vi "Find Average Center.vi"(5 "Position":i32, 7 "Tray Number":i32, 9 "XYZTheta":dbl[](array[numeric]), 11 "Gantry In":refnum<k24>) -> (1 "XYZTheta":dbl[](array[numeric]) format="%.6g", 3 "Gantry Out":refnum<k24>)   [LabVIEW 2021, in "Component Tray.lvclass"]
uses:
  Component Tray.lvclass
  Find Component.ctl
  Controller/Camera/Machine Vision.ctl
  C:/Program Files (x86)/Aerotech/A3200/LabVIEW/2010/Bin/Aerotech.A3200.dll
  Program Files (x86)/Aerotech/A3200/LabVIEW/2010/Bin/Aerotech.A3200.dll
  Controller/Camera/Image processing.ctl
  Controller/Camera/Camera settings.ctl
  Controller/Camera/Material.ctl
  Controller/Camera/Edmund Optics/Edmund Optics.lvclass
  C:/Users/HEP/Documents/GitHub/UCSB-Gantry-HEP/Classes/Controller/Camera/Camera.lvclass
  Program Files (x86)/National Instruments/LabVIEW 2021/examples/Connectivity/Python/support/PythonVersionsEnum.ctl
  Controller/Camera/Camera.lvclass
  Controller/Motion/A3200/A3200.lvclass
  Controller/Motion/Motion.lvclass
panel:
  out "Program Stopped":bool
  out "XY Graph":cluster{"X":dbl, "Y":dbl}[](graph)
  out "Sensor ID Location":dbl[](array[numeric])
  in  "Go to Sensor ID":bool
  out "CH1 Location":dbl[](array[numeric])
  in  "Verify CH1":bool
  out "CH1 correct?":bool
  in  "Go to CH1":bool
  in  "Focus step size":dbl format="%#_13g"
  in  "number of focus steps":i32
  out "Average Strength":dbl
  in  "Focus":bool
  in  "Material":T1
  out "All fiducials recorded":bool
  in  "Override presets":bool
  in  "Camera settings":T2={"Gamma"=1.6, "Gain"=0, "Sharpness"=0, "Contrast"=0.0, "Exposure"=0.0078125} {"Exposure" min=0.000244140625 max=0.5 scale=0.0002..0.5; "Contrast" min=0.0 max=1.0 scale=0.001..1.0; "Sharpness" min=0 max=2 step=1 scale=0.0..2.0; "Gain" min=0 max=100 step=1 scale=0.1..100.0; "Gamma" min=0.01 max=10.0 scale=0.01..10.0}
  in  "Image processing":T3={"Brightness"=128.0, "Contrast"=45.0, "Gamma"=1.0471123} {"Brightness" scale=0.0..400.0; "Contrast" scale=0.0..90.0; "Gamma" scale=0.005..5.0}
  in  "Machine Vision":T4
  out "Gantry":dbl[](array[numeric]) format="%.6g"
  out "Sum":dbl[](array[numeric]) format="%.6g"
  out "CH111/FD3 XY":dbl[](array[numeric]) format="%.6g"
  out "CH95/FD3 XY":dbl[](array[numeric]) format="%.6g"
  out "CH96/FD6 XY":dbl[](array[numeric]) format="%.6g"
  out "CH81/FD6 XY":dbl[](array[numeric]) format="%.6g"
  in  "Record CH95/FD3":bool
  in  "Record CH111/FD3":bool
  in  "Record CH96/FD6":bool
  in  "Record CH81/FD6":bool
  in  "Go to CH111/FD3":bool
  in  "Go to CH95/FD3":bool
  in  "Go to CH96/FD6":bool
  in  "Go to CH81/FD6":bool
  in  "Joystick":bool
  out "Camera":dbl[](array[numeric]) format="%.6g"
  in  "Go to Center":bool
  in  "Component":T5
  in  "Stop Program":bool
  out "Image":T6(plugin-control)
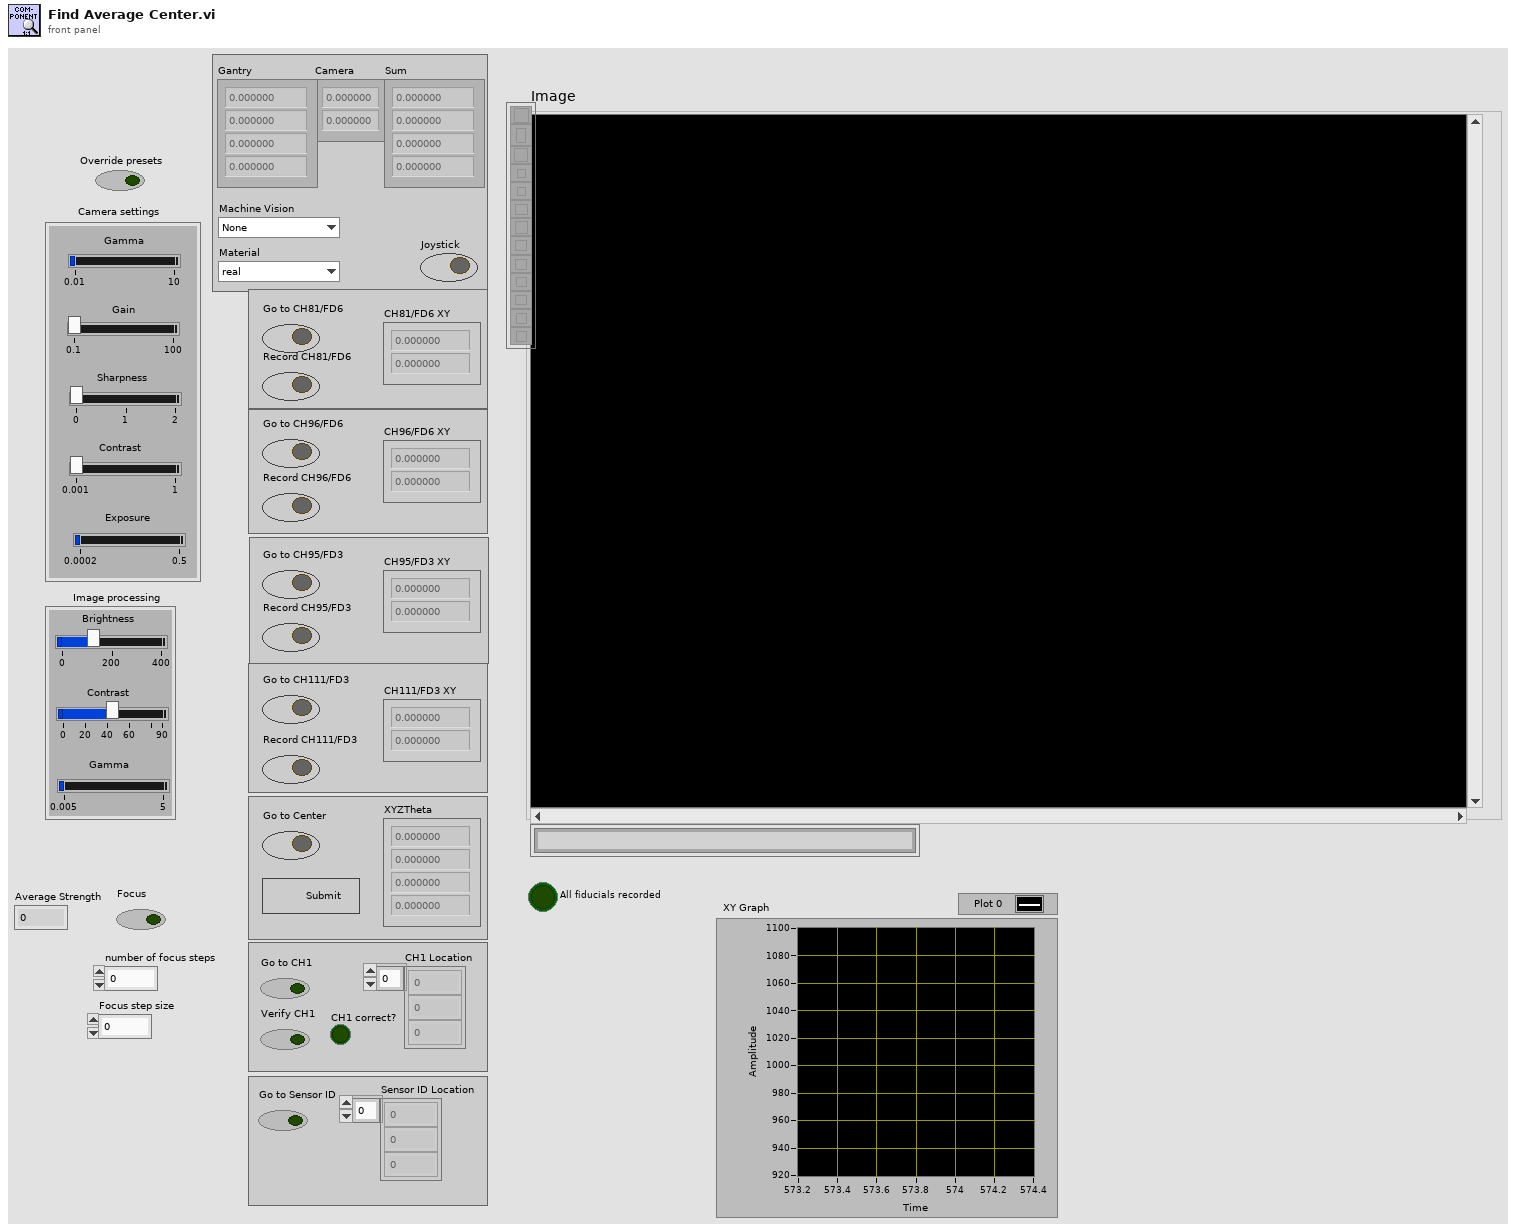
[diagram p1: front panel]
types:
  T1 = typedef "Camera.lvclass/Material.ctl" = enum16{"real", "dummy", "PETG"}
  T2 = typedef "Camera.lvclass/Camera settings.ctl" = cluster{"Gamma":dbl, "Gain":i64, "Sharpness":i64, "Contrast":dbl, "Exposure":dbl}
  T3 = typedef "Camera.lvclass/Image processing.ctl" = cluster{"Brightness":sgl, "Contrast":sgl, "Gamma":sgl}
  T4 = typedef "Camera.lvclass/Machine Vision.ctl" = enum16{"None", "Tray Fiducials", "HPK Silicon", "100um dot", "Hexaboard", "Corner (TL, BR)", "Corner (BL, TR)", "BP gold pad 1", "BP gold pad 2", "BP gold pad 3", "dummy sensor CH2", "dummy sensor CH7", "dummy sensor CH191", "dummy sensor CH197", "sensor box", "sensor circle", "PCB PETG CH2", "PCB PETG CH7", "PCB PETG CH191", "PCB PETG CH197"}
  T5 = typedef "Component Tray.lvclass/Find Component.ctl" = cluster{"New Fiducials":dbl[], "Past Fiducials":dbl[], "XYZTheta":dbl[], "Fiducials Path":path, "Position":i32, "CH1 Location":dbl[], "Sensor ID Location":dbl[]}
  T6 = typedef "IMAQ Image.ctl" = refnum<image>
  T7 = typedef "File Paths.ctl" = cluster{"Glue Pattern Folder":path, "Carrier Tray Folder":path, "Pick Up Tool Fixture Folder":path, "Components Folder":path, "Bellows Tool Offset.txt":path, "Pick Up Tool Offset.txt":path, "Dispense Tip Offset.txt":path, "Log Files":path, "Gantry Assembly Map.txt":path, "Syringe and offset map.txt":path, "Python DB Conn":path}
  T8 = typedef "PythonVersionsEnum.ctl" = enum16{"3.6", "3.7", "3.8", "3.9"}
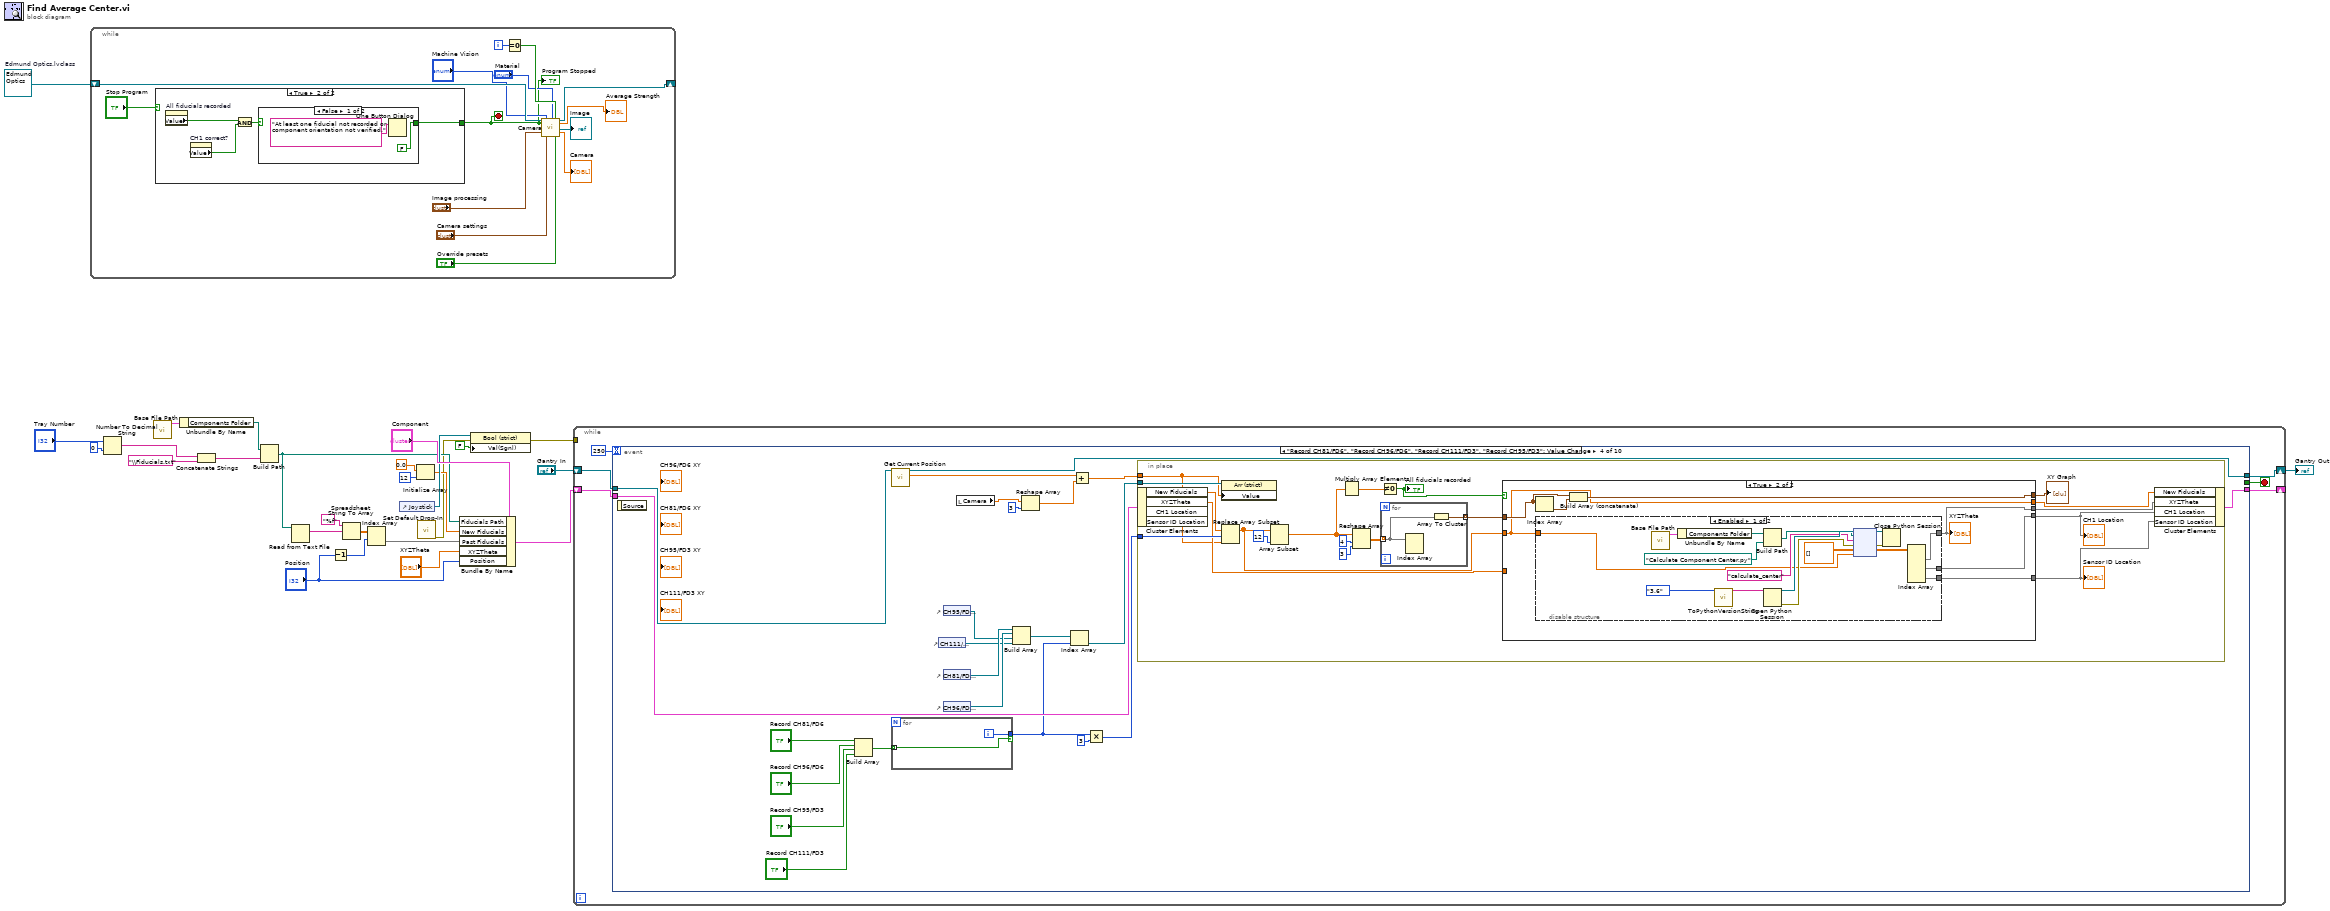
[diagram p0: block diagram]
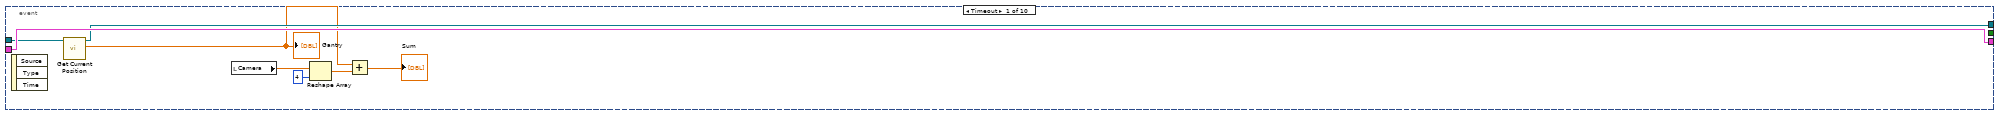
[diagram p2: hidden frame]
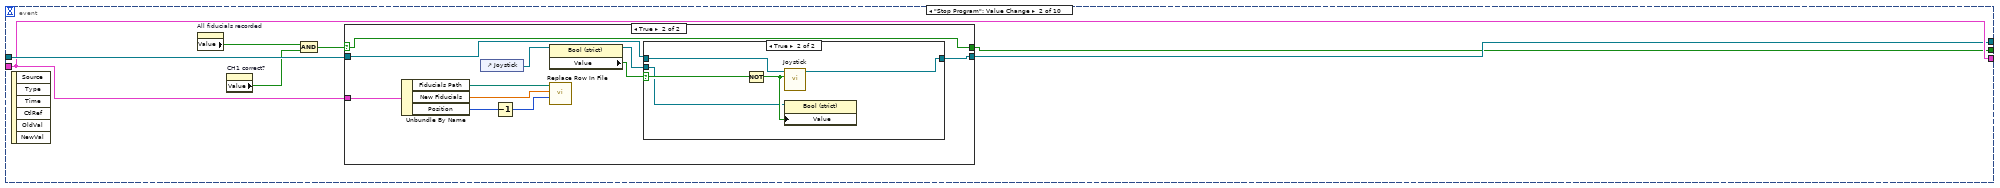
[diagram p3: hidden frame]
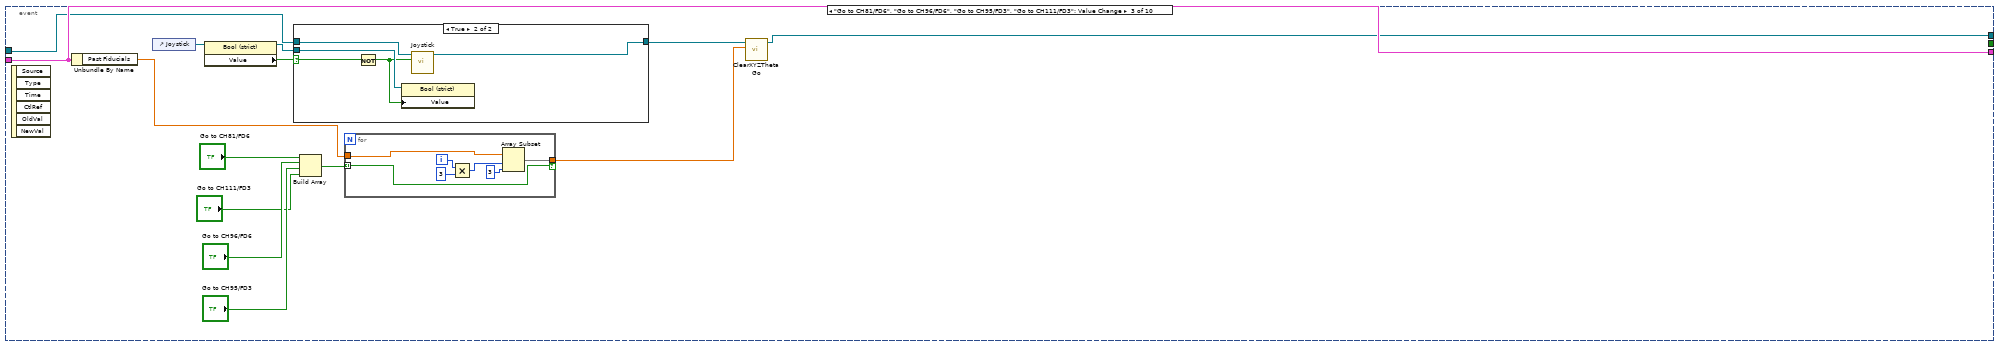
[diagram p6: hidden frame]
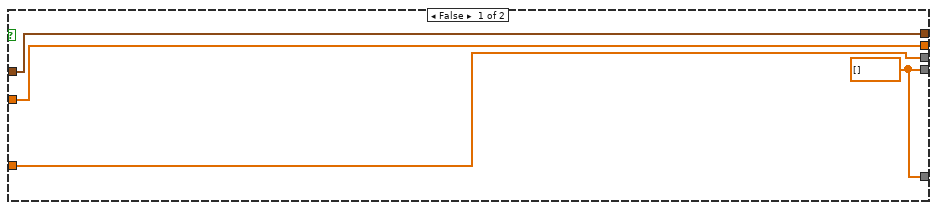
[diagram p8: hidden frame]
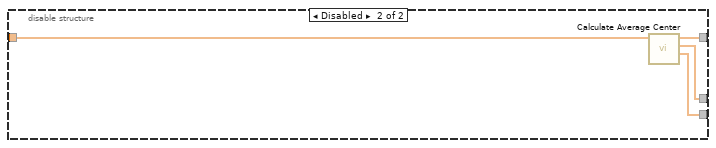
[diagram p9: hidden frame]
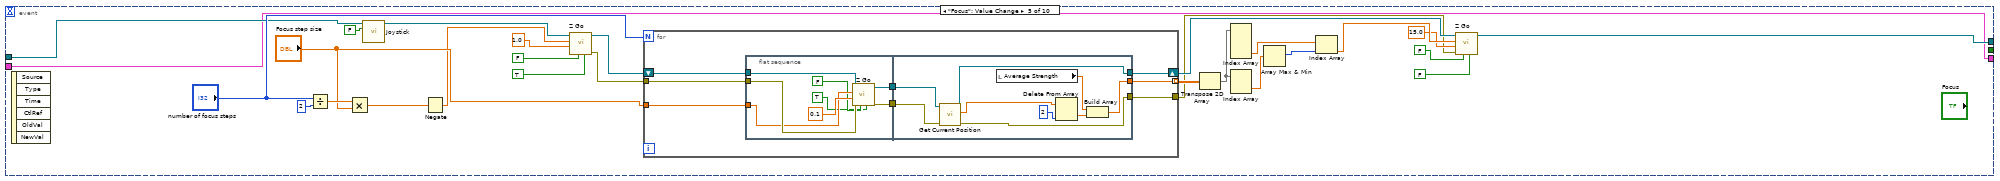
[diagram p10: hidden frame]
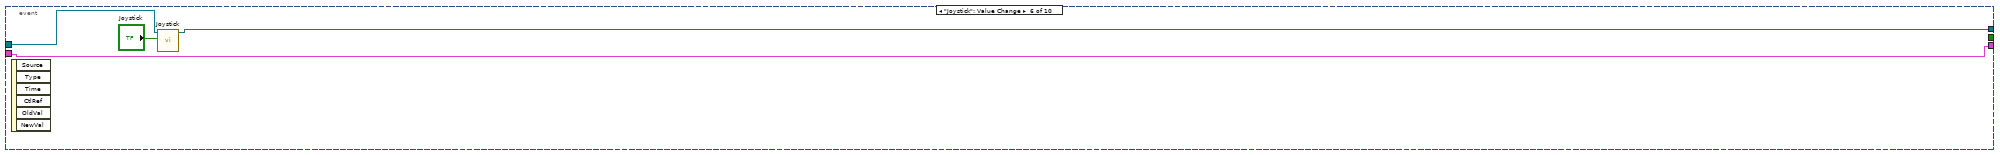
[diagram p11: hidden frame]
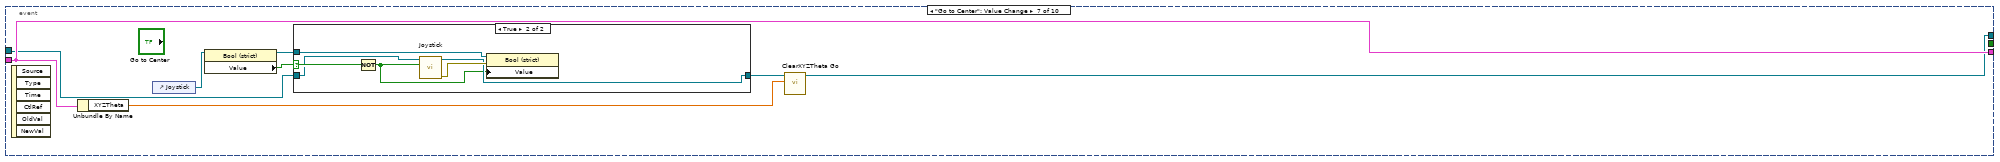
[diagram p12: hidden frame]
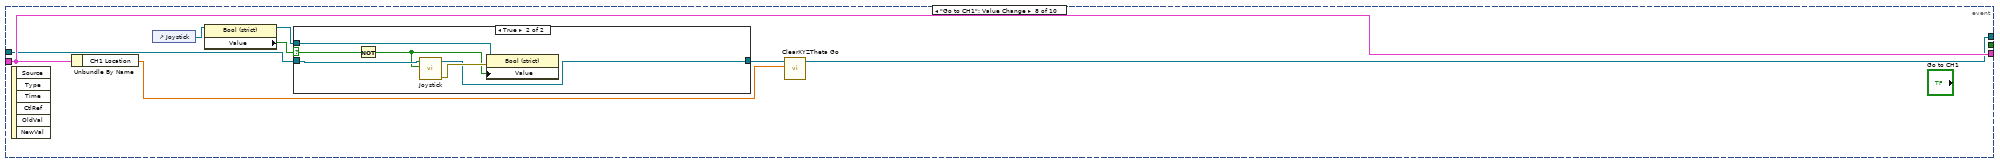
[diagram p14: hidden frame]
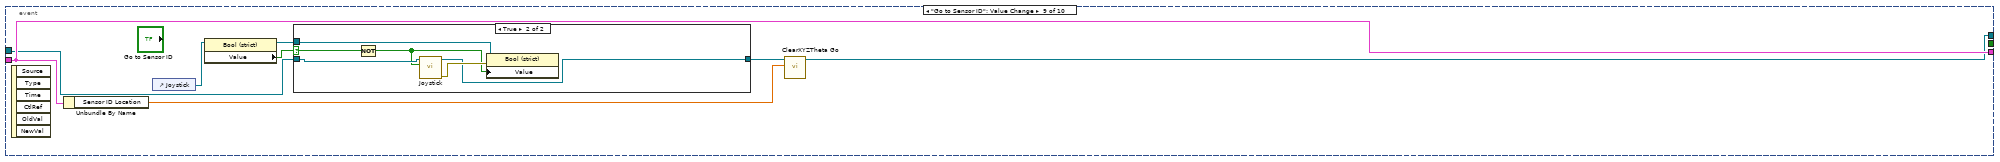
[diagram p16: hidden frame]
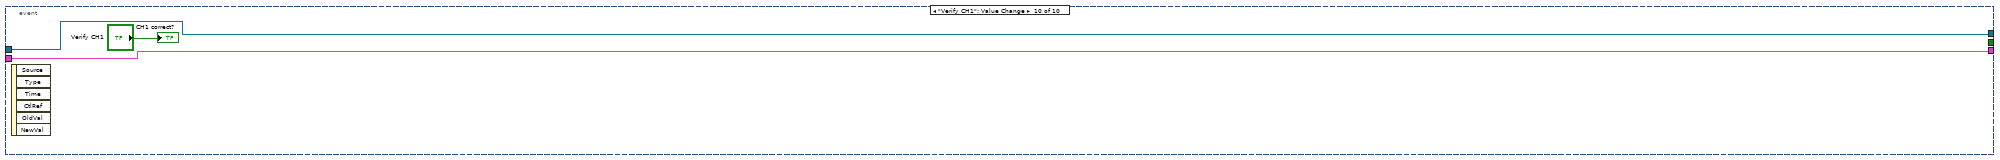
[diagram p18: hidden frame]
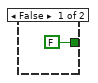
[diagram p19: hidden frame]
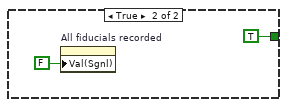
[diagram p20: hidden frame]
diagram:
  w22 = refnum<class "Edmund Optics.lvclass"> refnum  # Edmund Optics.lvclass
  n1 = while {
    shift-right: [w37] -> _
    shift-left: w22 -> [w41]
    i -> [w33]
    stop <- w28 stop-if-true
    n2 = case shown="True" "Stop Program" {
      tunnel: [FALSE w43] -> w28
      frame False {
      }
      frame True {
        n3 = property on="All fiducials recorded" class="Bool (strict)"() -> ("Value"=w46:bool)  [unwired: 2 in, 2 out]
        n4 = property on="CH1 correct?" class="Bool (strict)"() -> ("Value"=w44:bool)  [unwired: 2 in, 2 out]
        n5 = And(x=w46, y=w44) -> (x .and. y?=w45:bool)
        n6 = case shown="False" w45 {
          tunnel: [FALSE TRUE] -> w43
          frame False {
            n7 = One Button Dialog(message="At least one fiducial not recorded or component orientation not verified.") -> ()  [unwired: 1 in, 1 out]
          }
          frame True {
            n8 = property on="All fiducials recorded" class="Bool (strict)"("Val(Sgnl)"=FALSE) -> ()  [unwired: 2 in, 2 out]
          }
        }
      }
    }
    "Program Stopped" <- w28
    n9 = Equal To 0?(x=w33) -> (x = 0?=w32:bool)
    n10 = call "Camera.vi"("Camera in"=w41, "Stop"=w28, "BCG Image Processing"="Image processing", "Machine Vision"="Machine Vision", "Camera settings"="Camera settings", "Material"="Material", "Loop 0"=w32, "Override presets"="Override presets") -> ("Camera out"=w37:refnum<class "Edmund Optics.lvclass">, "Average Strength"=→"Average Strength":dbl, "Image"=→"Image":T6, "Camera"=→"Camera":dbl[])  [unwired: 5 in, 3 out]
  }
  n11 = Number To Decimal String(number="Tray Number", width (-)=i16 0) -> (decimal integer string=w16:string)
  n12 = call "Base File Path.vi"() -> ("Paths Out"=w13:T7)  [unwired: 11 in]
  n13 = Unbundle By Name(w13) -> ("Components Folder"=w15:path)
  n14 = Concatenate Strings(w16, "\\Fiducials.txt" ("string")) -> (w18:string)
  n15 = Build Path(base path=w15, name or relative path=w18) -> (appended path=w7:path)
  n16 = Read from Text File(file (use dialog)=w7) -> (text=w19:string)  [unwired: 3 in, 3 out]
  n17 = Decrement(x="Position") -> (x-1=w4:i32)
  n18 = Spreadsheet String To Array(format string="%f", spreadsheet string=w19) -> (array=w21:dbl[][])  [unwired: 2 in]
  n19 = Index Array(array=w21, index (row)=w4) -> (element=w11:dbl[])  [unwired: 1 in]
  n20 = control-ref of="Joystick"() -> (w25:refnum<vi>)
  n21 = Initialize Array(0.0 ("element"), 12 ("dimension size")) -> (w10:dbl[])
  n22 = call "Set Default Drop-In.vi"() -> ("error out"=w3:errorcluster)  [unwired: 11 in]
  n23 = Bundle By Name(cluster="Component", "Fiducials Path"=w7, "New Fiducials"=w10, "Past Fiducials"=w11, "XYZTheta"="XYZTheta", "Position"="Position") -> (w26:T5)
  n24 = property class="Bool (strict)"(reference=w25, error in=w3, "Val(Sgnl)"=FALSE) -> (error out=w23:errorcluster)  [unwired: 1 out]
  n25 = while {
    shift-right: [w54] -> _
    shift-left: w26 -> [w55]
    tunnel: w23 -> [_]
    shift-right: [w51] -> w1
    shift-left: "Gantry In" -> [w52]
    stop <- w56 stop-if-true
    n26 = event shown="[3] \"Record CH81/FD6\", \"Record CH96/FD6\", \"Record CH111/FD3\", \"Record CH95/FD3\": Value Change" {
      selector: _ -> [_ _ _ _ _ _ _ _ _ _]
      dyn-events: _ -> [_ _ _ _ _ _ _ _ _ _]
      timeout: 250 -> [_ _ _ _ _ _ _ _ _ _]
      tunnel: [_ w68 _ _ _ _ _ _ _ _] -> w56
      tunnel: w55 -> [w63 w70 w97 w140 w205 w251 w258 w273 w288 w298]
      tunnel: [w63 w70 w97 w139 w205 w251 w258 w273 w288 w298] -> w54
      tunnel: w52 -> [w59 w71 w94 w120 w207 w250 w254 w269 w284 w299]
      tunnel: [w58 w69 w91 w118 w206 w248 w252 w267 w282 w299] -> w51
      event Timeout {
        n27 = event-data() -> ()  [unwired: 1 in, 3 out]
        n28 = call "Get Current Position.vi"("Gantry In"=w59) -> ("XYZTheta Out"=w57:dbl[], "Gantry Out"=w58:refnum<k24>)  [unwired: 8 in, 1 out]
        "Gantry" <- w57
        n29 = local read "Camera"() -> (w62:dbl[])
        n30 = Reshape Array(w62, 4 ("dimension size")) -> (w60:dbl[])
        n31 = Add(x=w57, y=w60) -> (x+y=→"Sum":dbl[])
      }
      event "Stop Program": Value Change {
        n32 = event-data() -> ()  [unwired: 1 in, 6 out]
        n33 = property on="All fiducials recorded" class="Bool (strict)"() -> ("Value"=w66:bool)  [unwired: 2 in, 2 out]
        n34 = property on="CH1 correct?" class="Bool (strict)"() -> ("Value"=w67:bool)  [unwired: 2 in, 2 out]
        n35 = And(x=w66, y=w67) -> (x .and. y?=w65:bool)
        n36 = case shown="True" w65 {
          selector: w65 -> [w72 w81]
          tunnel: w71 -> [w73 w83]
          tunnel: w70 -> [_ w84]
          tunnel: [w73 w82] -> w69
          tunnel: [w72 w81] -> w68
          frame False {
          }
          frame True {
            n37 = Unbundle By Name(w84) -> ("Fiducials Path"=w78:path, "New Fiducials"=w77:dbl[], "Position"=w79:i32)
            n38 = control-ref of="Joystick"() -> (w75:refnum<vi>)
            n39 = Decrement(x=w79) -> (x-1=w80:i32)
            n40 = property class="Bool (strict)"(reference=w75) -> (reference out=w74:refnum<vi>, "Value"=w76:bool)  [unwired: 1 in, 1 out]
            n41 = call "Replace Row In File.vi"("Index"=w80, "Insert Array"=w77, "Path"=w78) -> ()  [unwired: 8 in, 1 out]
            n42 = case shown="True" w76 {
              selector: w76 -> [_ w90]
              tunnel: w83 -> [w85 w89]
              tunnel: [w85 w88] -> w82
              tunnel: w74 -> [_ w86]
              frame False {
              }
              frame True {
                n43 = Not(x=w90) -> (.not. x?=w87:bool)
                n44 = call "Joystick.vi"("Joystick"=w87, "Gantry In"=w89) -> ("Gantry Out"=w88:refnum<k24>)  [unwired: 8 in, 1 out]
                n45 = property class="Bool (strict)"(reference=w86, "Value"=w87) -> ()  [unwired: 1 in, 2 out]
              }
            }
          }
        }
      }
      event "Go to CH81/FD6", "Go to CH96/FD6", "Go to CH95/FD3", "Go to CH111/FD3": Value Change {
        n46 = event-data() -> ()  [unwired: 1 in, 6 out]
        n47 = Unbundle By Name(w97) -> ("Past Fiducials"=w99:dbl[])
        n48 = control-ref of="Joystick"() -> (w92:refnum<vi>)
        n49 = property class="Bool (strict)"(reference=w92) -> (reference out=w95:refnum<vi>, "Value"=w96:bool)  [unwired: 1 in, 1 out]
        n50 = case shown="True" w96 {
          selector: w96 -> [_ w110]
          tunnel: w94 -> [w105 w108]
          tunnel: [w105 w106] -> w93
          tunnel: w95 -> [_ w109]
          frame False {
          }
          frame True {
            n51 = Not(x=w110) -> (.not. x?=w107:bool)
            n52 = property class="Bool (strict)"(reference=w109, "Value"=w107) -> ()  [unwired: 1 in, 2 out]
            n53 = call "Joystick.vi"("Joystick"=w107, "Gantry In"=w108) -> ("Gantry Out"=w106:refnum<k24>)  [unwired: 8 in, 1 out]
          }
        }
        n54 = Build Array("Go to CH81/FD6", "Go to CH96/FD6", "Go to CH95/FD3", "Go to CH111/FD3") -> (w100:bool[])
        n55 = for {
          tunnel: w100 -> [w117] mode=indexing
          tunnel: w99 -> [w116]
          tunnel: [w111] -> w98 if=w117
          i -> [w114]
          n56 = Multiply(x=w114, y=3) -> (x*y=w112:i32)
          n57 = Array Subset(array=w116, index=w112, length=3) -> (w111:dbl[])
        }
        n58 = call "ClearXYZTheta Go.vi"("XYZTheta In"=w98, "Gantry In"=w93) -> ("Gantry Out"=w91:refnum<k24>)  [unwired: 7 in, 2 out]
      }
      event "Record CH81/FD6", "Record CH96/FD6", "Record CH111/FD3", "Record CH95/FD3": Value Change {
        n59 = event-data() -> ()  [unwired: 1 in, 1 out]
        n60 = Build Array("Record CH81/FD6", "Record CH96/FD6", "Record CH95/FD3", "Record CH111/FD3") -> (w134:bool[])
        n61 = call "Get Current Position.vi"("Gantry In"=w120) -> ("XYZTheta Out"=w119:dbl[], "Gantry Out"=w118:refnum<k24>)  [unwired: 8 in, 1 out]
        n62 = for {
          tunnel: w134 -> [w141] mode=indexing
          tunnel: [w142] -> w126 if=w141
          i -> [w142]
        }
        n63 = control-ref of="CH111/FD3 XY"() -> (w130:refnum<vi>)
        n64 = control-ref of="CH95/FD3 XY"() -> (w131:refnum<vi>)
        n65 = control-ref of="CH81/FD6 XY"() -> (w133:refnum<vi>)
        n66 = control-ref of="CH96/FD6 XY"() -> (w132:refnum<vi>)
        n67 = local read "Camera"() -> (w123:dbl[])
        n68 = Build Array(w133, w132, w131, w130) -> (w129:refnum<vi>[])
        n69 = Reshape Array(w123, 3 ("dimension size")) -> (w122:dbl[])
        n70 = Index Array(array=w129, index=w126) -> (element=w128:refnum<vi>)
        n71 = Add(x=w119, y=w122) -> (x+y=w121:dbl[])
        n72 = Multiply(x=w126, y=3) -> (x*y=w124:i32)
        n73 = in-place {
          in-place-border: w124 -> [w159]
          in-place-border: w128 -> [w157]
          in-place-border: w121 -> [w155]
          n74 = in-place-cluster #1(w140) -> ("New Fiducials"=w160:dbl[], "XYZTheta"=w156:dbl[])  [unwired: 2 out]
          n75 = property class="Arr (strict)"(reference=w157, "Value"=w155) -> ()  [unwired: 1 in, 2 out]
          n76 = Replace Array Subset(array=w160, new element=w155, index=w159) -> (w154:dbl[])
          n77 = Array Subset(array=w154, length=12) -> (w149:dbl[])  [unwired: 1 in]
          n78 = Multiply Array Elements(1:w149) -> (0:w152:dbl)
          n79 = Reshape Array(w149, 4 ("dimension size"), 3 ("dimension size")) -> (w146:dbl[][])
          n80 = Not Equal To 0?(x=w152) -> (x != 0?=w143:bool)
          "All fiducials recorded" <- w143
          n81 = for {
            tunnel: w146 -> [w162] mode=indexing
            tunnel: [w163] -> w145 mode=indexing
            n82 = Index Array(array=w162) -> ()  [unwired: 2 in, 2 out]
            n83 = Array To Cluster(array=w162) -> (cluster=w163:cluster{"[0]":dbl, "[1]":dbl})
          }
          n84 = case shown="True" w143 {
            tunnel: [w166 w168] -> w161
            tunnel: w154 -> [w167 w171]
            tunnel: [w167 w171] -> w158
            tunnel: w156 -> [w166 _]
            tunnel: [w165 w169] -> w151
            tunnel: [w165 w170] -> w150
            tunnel: w145 -> [w164 w174]
            tunnel: [w164 w172] -> w144
            frame False {
              w165 = dbl[] [] ("CH1 location")
            }
            frame True {
              n85 = Index Array(array=w174) -> (element=w173:cluster{"[0]":dbl, "[1]":dbl})  [unwired: 1 in]
              n86 = disable-structure shown="Enabled" {
                disable-tunnel: w171 -> [w179 w192]
                disable-tunnel: [w175 w195] -> w170
                disable-tunnel: [w176 w194] -> w169
                disable-tunnel: [w177 w193] -> w168
                frame Enabled {
                  n87 = call "Base File Path.vi"() -> ("Paths Out"=w184:T7)  [unwired: 11 in]
                  n88 = Unbundle By Name(w184) -> ("Components Folder"=w182:path)
                  n89 = call "ToPythonVersionString.vi"("python version"=PythonVersionsEnum."3.6") -> ("python version string"=w190:string)  [unwired: 10 in]
                  n90 = Build Path(base path=w182, name or relative path=path "Calculate Component Center.py") -> (appended path=w181:path)
                  n91 = Open Python Session(python version=w190) -> (session out=w189:refnum<k35>, error out=w187:errorcluster)  [unwired: 2 in]
                  n92 = node(w189, w181, "calculate_center" ("function name"), w187, dbl[][] [], w179) -> (w188:refnum<k35>, w186:errorcluster, w178:dbl[][])  [unwired: 1 in, 2 out]
                  n93 = Close Python Session(session in=w188, error in=w186) -> ()  [unwired: 1 out]
                  n94 = Index Array(array=w178) -> (element #1=w177:dbl[], element #2=w176:dbl[], element #3=w175:dbl[])  [unwired: 6 in]
                }
                frame Disabled {
                  n95 = call "Calculate Average Center.vi"("Gantry Fiducials"=w192) -> ("Sensor ID Location"=w195:dbl[], "CH1 Location"=w194:dbl[], "XYZTheta"=w193:dbl[])  [unwired: 8 in]
                }
              }
              "XYZTheta" <- w168
              n96 = Build Array (concatenate)(w174, w173) -> (w172:cluster{"[0]":dbl, "[1]":dbl}[])
            }
          }
          "CH1 Location" <- w151
          "Sensor ID Location" <- w150
          "XY Graph" <- w144
          n97 = in-place-cluster #1("New Fiducials"=w158, "XYZTheta"=w161, "CH1 Location"=w151, "Sensor ID Location"=w150) -> (w139:T5)
        }
      }
      event "Focus": Value Change {
        n98 = event-data() -> ()  [unwired: 1 in, 6 out]
        n99 = Divide(x="number of focus steps", y=2) -> (x/y=w210:dbl)
        n100 = Multiply(x=w210, y="Focus step size") -> (x*y=w208:dbl)
        n101 = call "Joystick.vi"("Joystick"=FALSE, "Gantry In"=w207) -> ("Gantry Out"=w201:refnum<k24>)  [unwired: 8 in, 1 out]
        n102 = Negate(x=w208) -> (-x=w202:dbl)
        n103 = call "Z Go.vi"("Increment"=TRUE, "Return Immediately"=FALSE ("Increment"), "Speed In"=1.0 ("Speed"), "Position In"=w202, "Gantry In"=w201) -> ("error out"=w199:errorcluster, "Gantry Out"=w200:refnum<k24>)  [unwired: 3 in, 2 out]
        n104 = for {
          N: "number of focus steps" -> [_]
          tunnel: [w227] -> w221 mode=indexing
          tunnel: w199 -> [w226]
          tunnel: [w224] -> w214
          shift-right: [w228] -> w215
          shift-left: w200 -> [w230]
          tunnel: "Focus step size" -> [w223]
          n105 = flat-sequence {
            tunnel: w230 -> [w238]
            tunnel: [w237] -> w229
            tunnel: w226 -> [w236]
            tunnel: [w235] -> w225
            tunnel: w223 -> [w233]
            tunnel: w229 -> [w247]
            tunnel: [w246] -> w228
            tunnel: [w245] -> w227
            tunnel: w225 -> [w241]
            tunnel: [w240] -> w224
            frame #0 {
              n106 = call "Z Go.vi"("Increment"=TRUE, "Return Immediately"=FALSE ("Increment"), "error in (no error)"=w236, "Speed In"=0.1 ("Speed"), "Position In"=w233, "Gantry In"=w238) -> ("error out"=w235:errorcluster, "Gantry Out"=w237:refnum<k24>)  [unwired: 2 in, 2 out]
            }
            frame #1 {
              n107 = call "Get Current Position.vi"("error in (no error)"=w241, "Gantry In"=w247) -> ("error out"=w240:errorcluster, "XYZTheta Out"=w244:dbl[], "Gantry Out"=w246:refnum<k24>)  [unwired: 7 in]
              n108 = local read "Average Strength"() -> (w239:dbl)
              n109 = Delete From Array(array=w244, index=2) -> (deleted portion=w242:dbl)  [unwired: 1 in, 1 out]
              n110 = Build Array(w239, w242) -> (w245:dbl[])
            }
          }
        }
        n111 = Transpose 2D Array(2D array=w221) -> (transposed array=w220:dbl[][])
        n112 = Index Array(array=w220) -> (element #2=w219:dbl[])  [unwired: 4 in, 1 out]
        n113 = Index Array(array=w220) -> (element=w222:dbl[])  [unwired: 2 in]
        n114 = Array Max & Min(array=w222) -> (max index (indices)=w218:i32)  [unwired: 3 out]
        n115 = Index Array(array=w219, index=w218) -> (element=w217:dbl)
        n116 = call "Z Go.vi"("Increment"=FALSE, "Return Immediately"=FALSE ("Increment"), "error in (no error)"=w214, "Speed In"=15.0 ("Speed"), "Position In"=w217, "Gantry In"=w215) -> ("Gantry Out"=w206:refnum<k24>)  [unwired: 2 in, 3 out]
      }
      event "Joystick": Value Change {
        n117 = event-data() -> ()  [unwired: 1 in, 6 out]
        n118 = call "Joystick.vi"("Joystick"="Joystick", "Gantry In"=w250) -> ("Gantry Out"=w248:refnum<k24>)  [unwired: 8 in, 1 out]
      }
      event "Go to Center": Value Change {
        n119 = event-data() -> ()  [unwired: 1 in, 6 out]
        n120 = Unbundle By Name(w258) -> ("XYZTheta"=w259:dbl[])
        n121 = control-ref of="Joystick"() -> (w255:refnum<vi>)
        n122 = property class="Bool (strict)"(reference=w255) -> (reference out=w256:refnum<vi>, "Value"=w257:bool)  [unwired: 1 in, 1 out]
        n123 = case shown="True" w257 {
          selector: w257 -> [_ w266]
          tunnel: w254 -> [w260 w263]
          tunnel: [w260 w262] -> w253
          tunnel: w256 -> [_ w265]
          frame False {
          }
          frame True {
            n124 = Not(x=w266) -> (.not. x?=w261:bool)
            n125 = call "Joystick.vi"("Joystick"=w261, "Gantry In"=w263) -> ("error out"=w264:errorcluster, "Gantry Out"=w262:refnum<k24>)  [unwired: 8 in]
            n126 = property class="Bool (strict)"(reference=w265, error in=w264, "Value"=w261) -> ()  [unwired: 2 out]
          }
        }
        n127 = call "ClearXYZTheta Go.vi"("XYZTheta In"=w259, "Gantry In"=w253) -> ("Gantry Out"=w252:refnum<k24>)  [unwired: 7 in, 2 out]
      }
      event "Go to CH1": Value Change {
        n128 = event-data() -> ()  [unwired: 1 in, 6 out]
        n129 = Unbundle By Name(w273) -> ("CH1 Location"=w274:dbl[])
        n130 = control-ref of="Joystick"() -> (w270:refnum<vi>)
        n131 = property class="Bool (strict)"(reference=w270) -> (reference out=w271:refnum<vi>, "Value"=w272:bool)  [unwired: 1 in, 1 out]
        n132 = case shown="True" w272 {
          selector: w272 -> [_ w281]
          tunnel: w269 -> [w275 w278]
          tunnel: [w275 w277] -> w268
          tunnel: w271 -> [_ w280]
          frame False {
          }
          frame True {
            n133 = Not(x=w281) -> (.not. x?=w276:bool)
            n134 = call "Joystick.vi"("Joystick"=w276, "Gantry In"=w278) -> ("error out"=w279:errorcluster, "Gantry Out"=w277:refnum<k24>)  [unwired: 8 in]
            n135 = property class="Bool (strict)"(reference=w280, error in=w279, "Value"=w276) -> ()  [unwired: 2 out]
          }
        }
        n136 = call "ClearXYZTheta Go.vi"("XYZTheta In"=w274, "Gantry In"=w268) -> ("Gantry Out"=w267:refnum<k24>)  [unwired: 7 in, 2 out]
      }
      event "Go to Sensor ID": Value Change {
        n137 = event-data() -> ()  [unwired: 1 in, 6 out]
        n138 = Unbundle By Name(w288) -> ("Sensor ID Location"=w289:dbl[])
        n139 = control-ref of="Joystick"() -> (w285:refnum<vi>)
        n140 = property class="Bool (strict)"(reference=w285) -> (reference out=w286:refnum<vi>, "Value"=w287:bool)  [unwired: 1 in, 1 out]
        n141 = case shown="True" w287 {
          selector: w287 -> [_ w296]
          tunnel: w284 -> [w290 w293]
          tunnel: [w290 w292] -> w283
          tunnel: w286 -> [_ w295]
          frame False {
          }
          frame True {
            n142 = Not(x=w296) -> (.not. x?=w291:bool)
            n143 = call "Joystick.vi"("Joystick"=w291, "Gantry In"=w293) -> ("error out"=w294:errorcluster, "Gantry Out"=w292:refnum<k24>)  [unwired: 8 in]
            n144 = property class="Bool (strict)"(reference=w295, error in=w294, "Value"=w291) -> ()  [unwired: 2 out]
          }
        }
        n145 = call "ClearXYZTheta Go.vi"("XYZTheta In"=w289, "Gantry In"=w283) -> ("Gantry Out"=w282:refnum<k24>)  [unwired: 7 in, 2 out]
      }
      event "Verify CH1": Value Change {
        n146 = event-data() -> ()  [unwired: 1 in, 6 out]
        "CH1 correct?" <- "Verify CH1"
      }
    }
  }
  "Gantry Out" <- w1
